vi "Extract datatype from parameters JSON.vi"(0 "parameters JSON in":string, 11 "error in (no error)":errorcluster) -> (4 "datatype enum":T1, 6 "datatype valid?":bool, 8 "datatype string":string, 15 "error out":errorcluster)   [LabVIEW 2019, in "mmW_commands.lvlib"]
uses:
  mmW_commands.lvlib
  <vilib>/addons/_JKI.lib/Serialization/JSON/JKI JSON Serialization.lvlib
  commands/typedefs/datatypes_.ctl
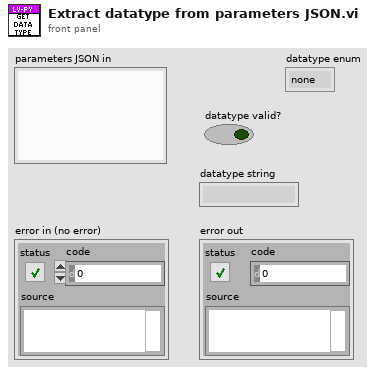
[diagram p1: front panel]
types:
  T1 = typedef "mmW_commands.lvlib/datatypes_.ctl" = enum16{"none", "string", "interleaved_I16", "interleaved_I32", "I16_array", "I32_array"}
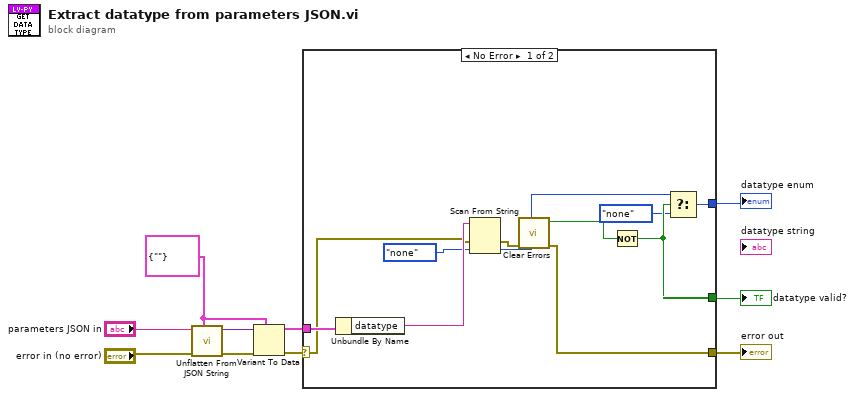
[diagram p0: block diagram]
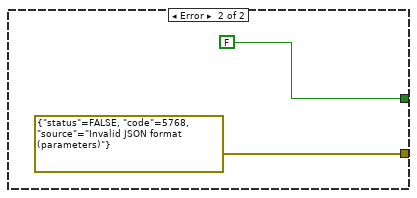
[diagram p2: hidden frame]
diagram:
  w4 = cluster{"datatype":string} {"datatype"=""}
  n1 = call <vilib>:"Unflatten From JSON String.vi"("Type and Defaults"=w4, "error in (no error)"="error in (no error)", "JSON String"="parameters JSON in") -> ("error out"=w7:errorcluster, "Variant"=w5:variant)  [unwired: 7 in]
  n2 = Variant To Data(error in=w7, type=w4, Variant=w5) -> (data=w6:cluster{"datatype":string}, error out=w8:errorcluster)
  n3 = case shown="No Error" w8 {
    selector: w8 -> [w12 _]
    tunnel: w6 -> [w21 _]
    tunnel: [w14 FALSE] -> w10
    tunnel: [w11 errorcluster {"status"=FALSE, "code"=5768, "source"="Invalid JSON format (parameters)"} ("error IO")] -> w9
    tunnel: [w20 _] -> w1
    frame No Error {
      n4 = Unbundle By Name(w21) -> ("datatype"=w19:string)
      n5 = Scan From String(input string=w19, error in=w12, default 1=datatypes_."none" ("datatype enum")) -> (error out=w16:errorcluster, output 1=w17:T1)  [unwired: 2 in, 2 out]
      n6 = call <vilib>:"Clear Errors.vi"("error in (no error)"=w16) -> ("error out"=w11:errorcluster, "specific error cleared?"=w15:bool)  [unwired: 5 in]
      n7 = Not(x=w15) -> (.not. x?=w14:bool)
      n8 = Select(t=w17, s=w14, f=datatypes_."none") -> (s? t:f=w20:T1)
    }
    frame Error {
    }
  }
  "datatype enum" <- w1
  "datatype valid?" <- w10
  "error out" <- w9
